vi "Read Icon (BitMap).vi"(8 "error in (no error)":errorcluster, 11 "Control in":refnum<class "Control.lvclass">) -> (0 "error out":errorcluster, 1 "Icon (BitMap) True":refnum<class "BitMap.lvclass">, 2 "Icon (BitMap) False":refnum<class "BitMap.lvclass">, 3 "Control out":refnum<class "Control.lvclass">)   [LabVIEW 2012, in "Control.lvclass"]
uses:
  Control.lvclass
  <userlib>/BitMan/BitMap class/BitMap.lvclass
  Control.lvclass/Control.ctl
  <userlib>/BitMan/Built-in Filters class/Built-in Filters.lvclass
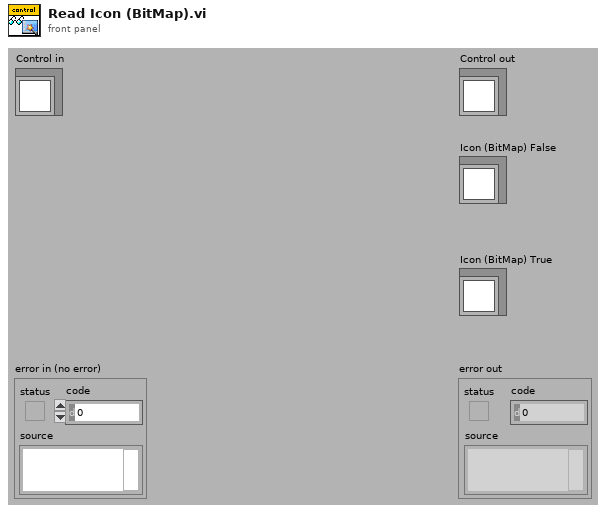
[diagram p1: front panel]
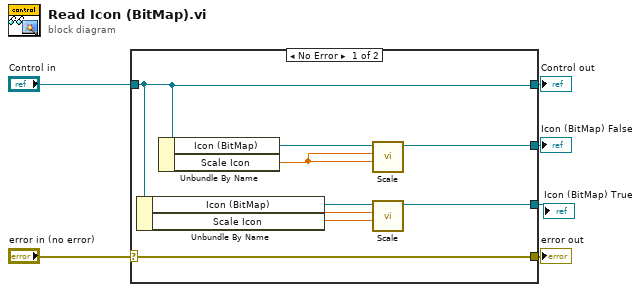
[diagram p0: block diagram]
diagram:
  n1 = case shown="No Error" "error in (no error)" {
    selector: "error in (no error)" -> [w14 w15]
    tunnel: [w14 w15] -> w5
    tunnel: [w8 w16] -> w3
    tunnel: "Control in" -> [w8 w16]
    tunnel: [w12 _] -> w2
    tunnel: [w7 _] -> w1
    frame No Error {
      n2 = Unbundle By Name(w8) -> ("Icon (BitMap)"=w9:refnum<class "BitMap.lvclass">, "Scale Icon"=w10:dbl)
      n3 = Unbundle By Name(w8) -> ("Icon (BitMap)"=w13:refnum<class "BitMap.lvclass">, "Scale Icon"=w11:dbl)
      n4 = call <userlib>:"Scale.vi"("y"=w11, "x"=w11, "Bitmap in (optional)"=w13) -> ("Bitmap out"=w12:refnum<class "BitMap.lvclass">)  [unwired: 3 in, 5 out]
      n5 = call <userlib>:"Scale.vi"("y"=w10, "x"=w10, "Bitmap in (optional)"=w9) -> ("Bitmap out"=w7:refnum<class "BitMap.lvclass">)  [unwired: 3 in, 5 out]
    }
    frame Error {
    }
  }
  "error out" <- w5
  "Control out" <- w3
  "Icon (BitMap) False" <- w2
  "Icon (BitMap) True" <- w1
